vi "QD_Backend_Module.vi"(0 "State_and_Data_In":T1, 1 "Max_Queue_Size_In":i32=-1, 2 "Queue_Name_In":string, 5 "State_and_Data_N_In":T1[](array[typedef]), 7 "Time_Out_In_ms (-1)":i32, 11 "Error_In":errorcluster, 13 "Queue_Operation":T2=enum."Dequeue") -> (4 "State_and_Data_Out":T1={"State"="FP_Update", "Data"=variant(cluster{"Current_Data":dbl, "Temp_Data":dbl} {"Current_Data"=0.0, "Temp_Data"=0.0})}, 6 "State_and_Data_N_Out":T1[](array[typedef]), 15 "Error_Out":errorcluster)   [LabVIEW 2021]
doc: "Used to transfer data from one vi to another using queue."
uses:
  Controls/State_and_Data.ctl
  Controls/Queue_Operation_Select.ctl
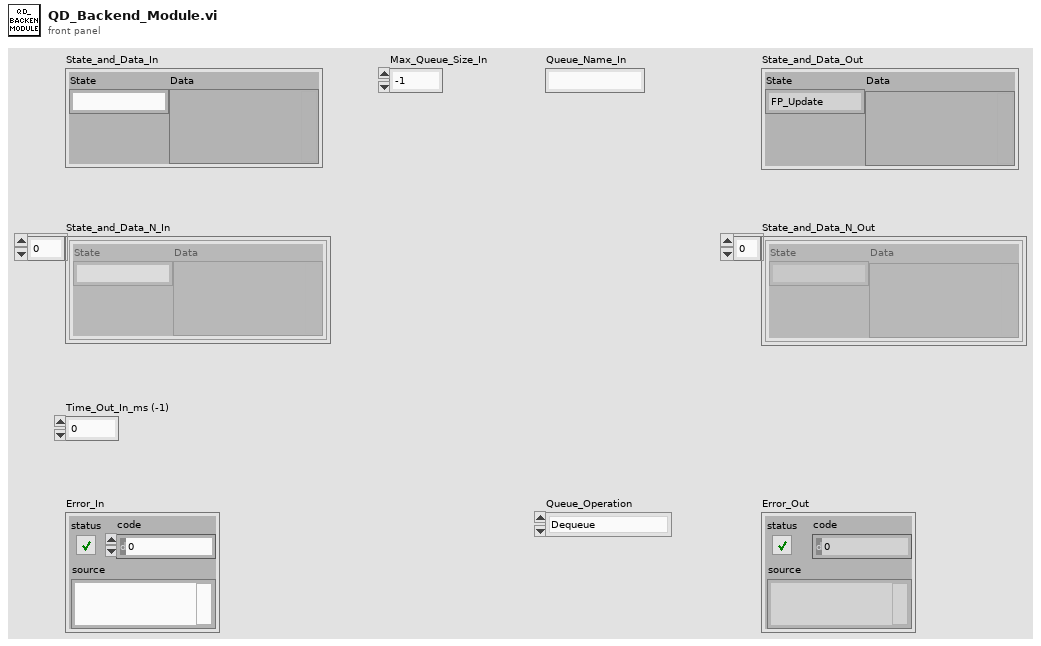
[diagram p1: front panel]
types:
  T1 = typedef "State_and_Data.ctl" = cluster{"State":string, "Data":variant}
  T2 = typedef "Queue_Operation_Select.ctl" = enum16{"Obtain_Queue", "Enqueue", "Enqueue_First", "Enqueue_N", "Lossy_Enqueue", "Preview", "Queue_Status", "Dequeue", "Flush", "Release_Queue"}
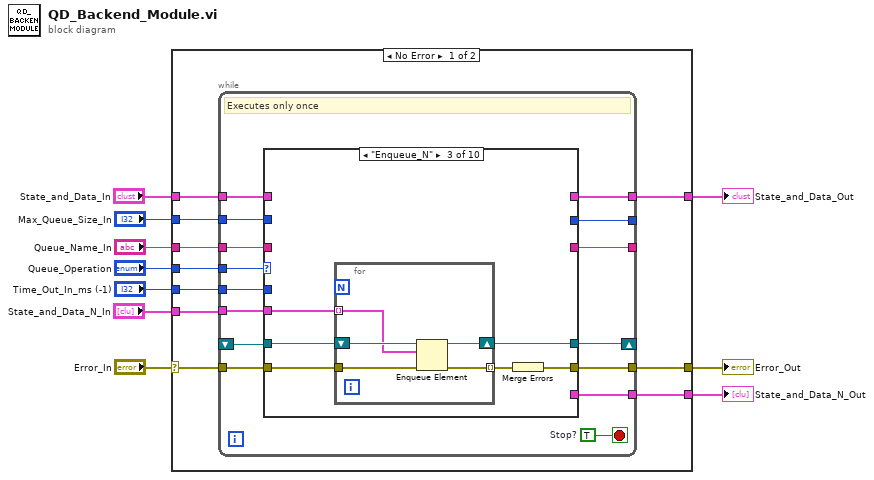
[diagram p0: block diagram]
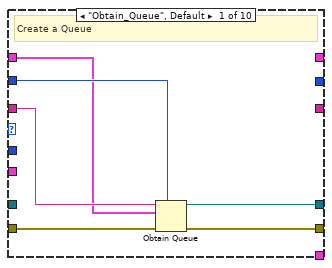
[diagram p2: hidden frame]
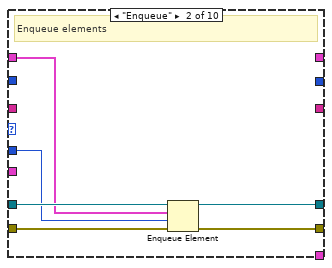
[diagram p3: hidden frame]
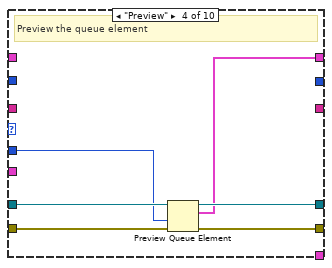
[diagram p4: hidden frame]
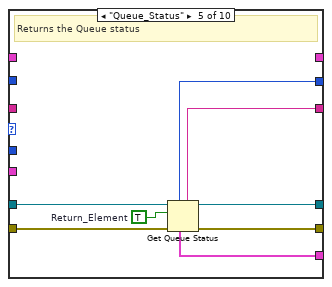
[diagram p5: hidden frame]
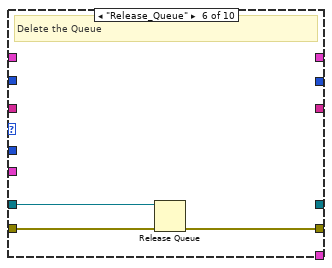
[diagram p6: hidden frame]
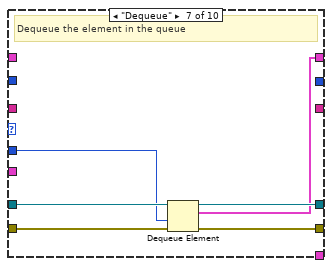
[diagram p7: hidden frame]
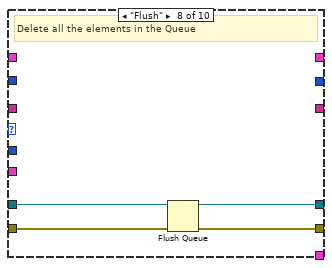
[diagram p8: hidden frame]
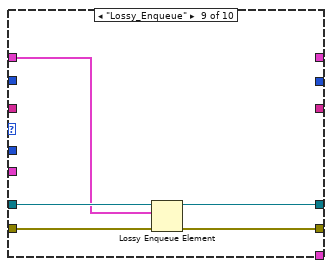
[diagram p9: hidden frame]
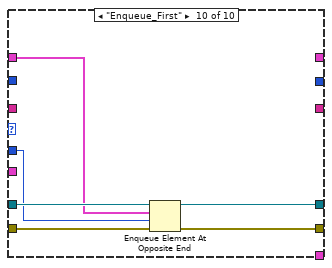
[diagram p10: hidden frame]
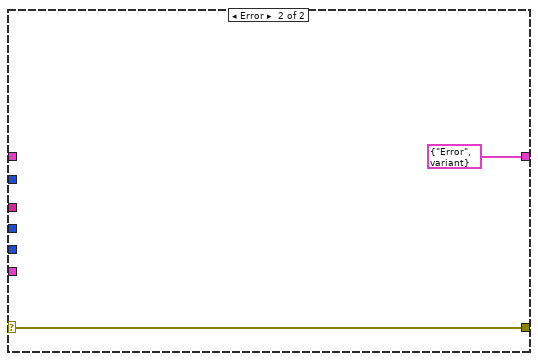
[diagram p11: hidden frame]
diagram:
  n1 = case shown="No Error" "Error_In" {
    selector: "Error_In" -> [w11 w98]
    tunnel: "Max_Queue_Size_In" -> [w20 _]
    tunnel: [w19 w98] -> w9
    tunnel: "Time_Out_In_ms (-1)" -> [w18 _]
    tunnel: "Queue_Operation" -> [w17 _]
    tunnel: "Queue_Name_In" -> [w16 _]
    tunnel: "State_and_Data_In" -> [w15 _]
    tunnel: [w14 T1 {"State"="Error", "Data"=variant} ("State_and_Data_In")] -> w4
    tunnel: [w13 _] -> w3
    tunnel: "State_and_Data_N_In" -> [w12 _]
    frame No Error {
      n2 = while {
        tunnel: w20 -> [w35]
        tunnel: w18 -> [w32]
        tunnel: [w30] -> _
        tunnel: w17 -> [w27]
        tunnel: [w25] -> w13
        shift-right: [w28] -> _
        shift-left: _ -> [w23]
        tunnel: w11 -> [w24]
        tunnel: [w34] -> w19
        tunnel: w12 -> [w21]
        tunnel: w16 -> [w26]
        tunnel: [w29] -> _
        tunnel: w15 -> [w33]
        tunnel: [w31] -> w14
        stop <- w22 stop-if-true
        w22 = TRUE  # Stop?
        # "Executes only once"
        n3 = case shown="\"Enqueue_N\"" w27 {
          tunnel: w24 -> [w41 w47 w53 w63 w71 w74 w80 w84 w89 w96]
          tunnel: w26 -> [w39 _ _ _ _ _ _ _ _ _]
          tunnel: w35 -> [w38 _ _ _ _ _ _ _ _ _]
          tunnel: [w36 w43 w50 w62 w70 _ w79 w83 w88 w93] -> w28
          tunnel: [w40 w46 w48 w61 w69 w73 w77 w82 w87 w95] -> w34
          tunnel: w23 -> [_ w45 w51 w64 w72 w75 w81 w85 w90 w94]
          tunnel: w33 -> [w37 w44 _ _ _ _ _ _ w86 w92]
          tunnel: w32 -> [_ w42 _ w60 _ _ w76 _ _ w91]
          tunnel: [_ _ _ w59 _ _ w78 _ _ _] -> w31
          tunnel: [_ _ _ _ w68 _ _ _ _ _] -> w30
          tunnel: [_ _ _ _ w67 _ _ _ _ _] -> w29
          tunnel: [_ _ _ _ w66 _ _ _ _ _] -> w25
          tunnel: w21 -> [_ _ w49 _ _ _ _ _ _ _]
          frame "Obtain_Queue", Default {
            # "Create a Queue"
            n4 = Obtain Queue(max queue size (-1, unlimited)=w38, name (unnamed)=w39, element data type=w37, error in (no error)=w41) -> (queue out=w36:refnum<queue>, error out=w40:errorcluster)  [unwired: 1 in, 1 out]
          }
          frame "Enqueue" {
            # "Enqueue elements"
            n5 = Enqueue Element(queue=w45, element=w44, timeout in ms (-1)=w42, error in (no error)=w47) -> (queue out=w43:refnum<queue>, error out=w46:errorcluster)  [unwired: 1 out]
          }
          frame "Enqueue_N" {
            n6 = for {
              tunnel: w49 -> [w54] mode=indexing
              tunnel: w53 -> [w58]
              tunnel: [w57] -> w52 mode=indexing
              shift-right: [w55] -> w50
              shift-left: w51 -> [w56]
              n7 = Enqueue Element(queue=w56, element=w54, error in (no error)=w58) -> (queue out=w55:refnum<queue>, error out=w57:errorcluster)  [unwired: 1 in, 1 out]
            }
            n8 = Merge Errors(w52) -> (w48:errorcluster)
          }
          frame "Preview" {
            # "Preview the queue element"
            n9 = Preview Queue Element(queue=w64, timeout in ms (-1)=w60, error in (no error)=w63) -> (queue out=w62:refnum<queue>, element=w59:T1, error out=w61:errorcluster)  [unwired: 1 out]
          }
          frame "Queue_Status" {
            w65 = TRUE  # Return_Element
            # "Returns the Queue status"
            n10 = Get Queue Status(queue=w72, return elements? (F)=w65, error in (no error)=w71) -> (queue out=w70:refnum<queue>, queue name=w67:string, max queue size=w68:i32, error out=w69:errorcluster, elements=w66:T1[])  [unwired: 3 out]
          }
          frame "Release_Queue" {
            # "Delete the Queue"
            n11 = Release Queue(queue=w75, error in (no error)=w74) -> (error out=w73:errorcluster)  [unwired: 1 in, 2 out]
          }
          frame "Dequeue" {
            # "Dequeue the element in the queue"
            n12 = Dequeue Element(queue=w81, timeout in ms (-1)=w76, error in (no error)=w80) -> (queue out=w79:refnum<queue>, element=w78:T1, error out=w77:errorcluster)  [unwired: 1 out]
          }
          frame "Flush" {
            # "Delete all the elements in the Queue"
            n13 = Flush Queue(queue=w85, error in (no error)=w84) -> (queue out=w83:refnum<queue>, error out=w82:errorcluster)  [unwired: 1 out]
          }
          frame "Lossy_Enqueue" {
            n14 = Lossy Enqueue Element(queue=w90, element=w86, error in (no error)=w89) -> (queue out=w88:refnum<queue>, error out=w87:errorcluster)  [unwired: 2 out]
          }
          frame "Enqueue_First" {
            n15 = Enqueue Element At Opposite End(queue=w94, element=w92, timeout in ms (-1)=w91, error in (no error)=w96) -> (queue out=w93:refnum<queue>, error out=w95:errorcluster)  [unwired: 1 out]
          }
        }
      }
    }
    frame Error {
    }
  }
  "Error_Out" <- w9
  "State_and_Data_Out" <- w4
  "State_and_Data_N_Out" <- w3
